vi "WM Stroke to Wave Height.vi"(1 "Paddle Height (m)":dbl=3.3147 format="%.2f", 2 "Wave Period (s)":dbl format="%.2f", 3 "Water Depth (m)":dbl step=0.01 format="%.2f", 4 "Flap Amplitude from x=0 (m)":dbl format="%.2f") -> (0 "Wave Height (m)":dbl format="%.2f")   [LabVIEW 2012]
panel:
  # "Flap Stroke at Water line (S)"
  # "Flap Amplitude From x=0 (A')"
  # "Total Flap Stroke (S')"
  # "Flap Height (h')"
  # "Wave Height (Peak to trough) (H)"
  # "Wave Amplitude (z=0 to Peak) (A)"
  # "Wave Height to Flap Stroke at Water Line ( [H/S] )"
  # "Water Depth (h)"
  # "H = 2 * h * [H/S] *A' / h'"
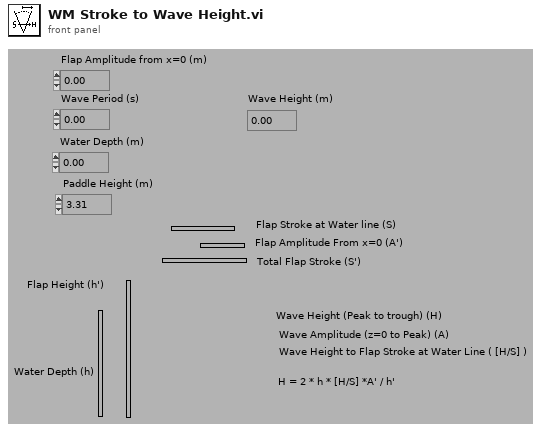
[diagram p1: front panel]
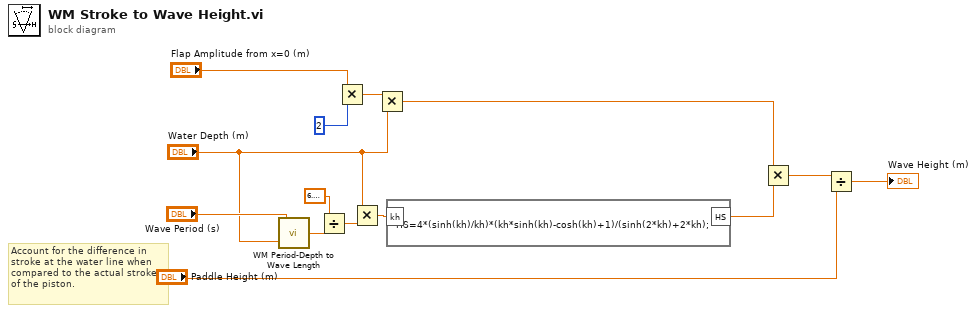
[diagram p0: block diagram]
diagram:
  # "Account for the difference in \nstroke at the water line when \ncompared to the actual stroke\nof the piston."
  n1 = call "WM Period-Depth to Wave Length.vi"("Water Depth"="Water Depth (m)", "Period"="Wave Period (s)") -> ("WaveLength"=w13:dbl)
  n2 = Divide(x=6.283185307179586, y=w13) -> (x/y=w12:dbl)
  n3 = Multiply(x="Flap Amplitude from x=0 (m)", y=2) -> (x*y=w8:dbl)
  n4 = Multiply(x="Water Depth (m)", y=w12) -> (x*y=w11:dbl)
  n5 = Multiply(x=w8, y="Water Depth (m)") -> (x*y=w6:dbl)
  n6 = formula code="HS=4*(sinh(kh)/kh)*(kh*sinh(kh)-cosh(kh)+1)/(sinh(2*kh)+2*kh);"("kh"=w11) -> ("HS"=w7:dbl)
  n7 = Multiply(x=w6, y=w7) -> (x*y=w2:dbl)
  n8 = Divide(x=w2, y="Paddle Height (m)") -> (x/y=→"Wave Height (m)":dbl)
